vi "niRFUtil TRC Waveform to Trace (complex wfm).vi"(7 "Complex Waveform":T2 {"y" format="%.2f"; "dx" format="%^.2e"; "x0" format="%^.2e"}) -> (8 "Measurement Trace":T1 format="%.2f")   [LabVIEW 2015, in "niRFUtil.lvlib"]
doc: "(c) Copyright 2006, National Instruments, Inc. This VI may not be duplicated, sold, or distributed without written consent from National Instruments."
uses:
  niRFUtil.lvlib
  Includes/niRFUtil INC Complex Waveform.ctl
  Includes/niRFUtil INC Complex Array.ctl
  Includes/niRFUtil INC Trace.ctl
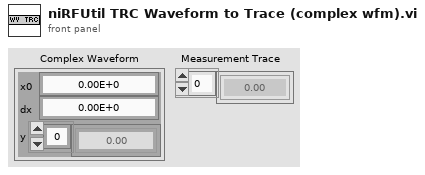
[diagram p1: front panel]
types:
  T1 = typedef "niRFUtil.lvlib/niRFUtil INC Trace.ctl" = sgl[]
  T2 = typedef "niRFUtil.lvlib/niRFUtil INC Complex Waveform.ctl" = cluster{"x0":dbl, "dx":dbl, "y":T3}
  T3 = typedef "niRFUtil.lvlib/niRFUtil INC Complex Array.ctl" = csg[]
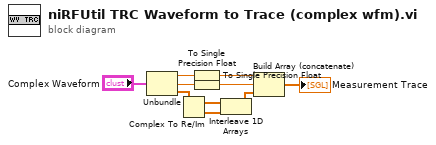
[diagram p0: block diagram]
diagram:
  n1 = Unbundle("Complex Waveform") -> ("x0"=w6:dbl, "dx"=w5:dbl, "y"=w7:T3)
  n2 = Complex To Re/Im(x + iy=w7) -> (x=w8:sgl[], y=w9:sgl[])
  n3 = To Single Precision Float(number=w6) -> (single precision float=w2:sgl)
  n4 = To Single Precision Float(number=w5) -> (single precision float=w1:sgl)
  n5 = Interleave 1D Arrays(w8, w9) -> (w4:sgl[])
  n6 = Build Array (concatenate)(w2, w1, w4) -> (→"Measurement Trace":sgl[])
